vi "AdafruitSeesawNeoPixel.vi"() -> ()   [LabVIEW 2020, in "CTI-Scratchpad.lvlib"]
uses:
  CTI-Scratchpad.lvlib
  CTI/Identity.ctl
  AdafruitSeeSaw/NeoPixelRingPatterns.ctl
  CTI/Error Reporting.ctl
  CTI/I2C Address.ctl
  CTI/GPIO Number.ctl
  CTI/I2C Number.ctl
  CTI/Session/Session.lvclass
  CTI/VisaComms/VisaComms.lvclass
  CTI/CTI.lvlib
  CTI-Peripheral/AdaFruit-Seesaw/AdaFruit-Seesaw.lvclass
panel:
  in  "Timeout":i32=100
  in  "Patterns":T1=enum."ColorWipe"
  in  "Colour Set":T2={"Color Box 0"=16711803, "Color Box 1"=6618880, "Color Box 2"=16716496, "Color Box 4"=9567230, "Color Box 5"=6618880, "Color Box 6"=3381759, "Color Box 7"=9567230, "Color Box 8"=6618880, "Color Box 9"=16860, "Color Box 10"=6618880, "Color Box 11"=6618880, "Color Box 12"=6618880}
  out "NeoPixel Ring":T3={"Color Box"=0, "Color Box 2"=0, "Color Box 3"=0, "Color Box 4"=0, "Color Box 5"=0, "Color Box 6"=0, "Color Box 7"=0, "Color Box 8"=0, "Color Box 9"=0, "Color Box 10"=0, "Color Box 11"=16711680, "Color Box 12"=16777228}
  in  "Brightness":u8=5
  out "loop":i32=14774
  out "Identity":T4
  in  "Grove Connector":enum16{"I2C0", "I2C1"}(ring)
  in  "Port":refnum<visa-resource-name>="COM11"
  out "error out 2":errorcluster
  in  "Stop":bool
  out "error out":errorcluster
  # "https://www.adafruit.com/product/1643"
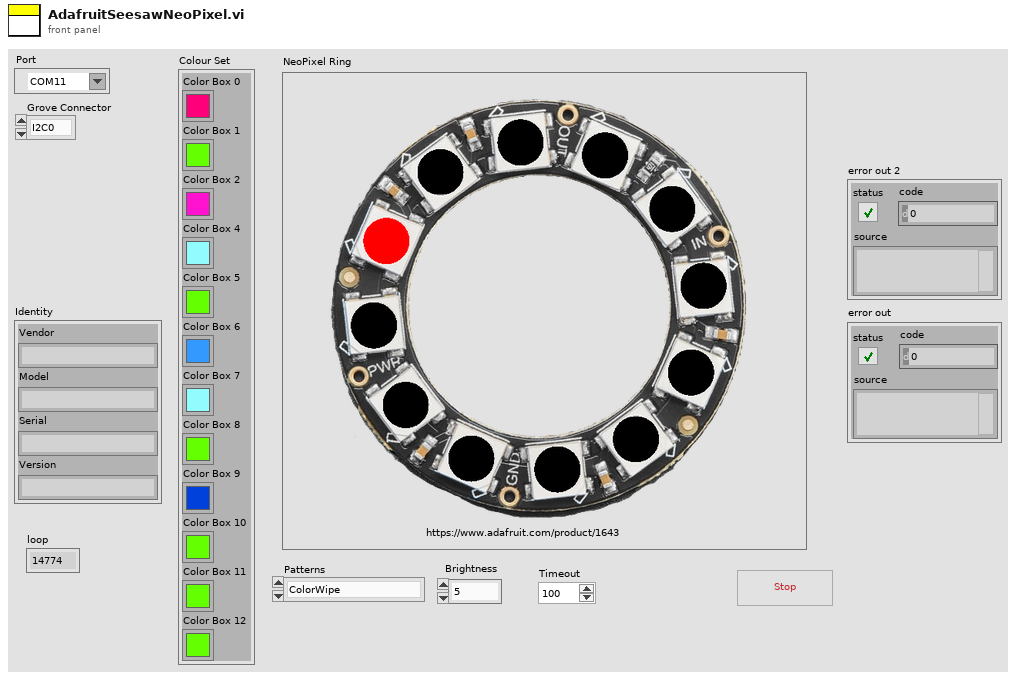
[diagram p1: front panel]
types:
  T1 = typedef "CTI-Scratchpad.lvlib/NeoPixelRingPatterns.ctl" = enum16{"Set Colour", "ColorWipe", "TheatreChase", "Rainbow"}
  T2 = cluster{"Color Box 0":u32, "Color Box 1":u32, "Color Box 2":u32, "Color Box 4":u32, "Color Box 5":u32, "Color Box 6":u32, "Color Box 7":u32, "Color Box 8":u32, "Color Box 9":u32, "Color Box 10":u32, "Color Box 11":u32, "Color Box 12":u32}
  T3 = cluster{"Color Box":u32, "Color Box 2":u32, "Color Box 3":u32, "Color Box 4":u32, "Color Box 5":u32, "Color Box 6":u32, "Color Box 7":u32, "Color Box 8":u32, "Color Box 9":u32, "Color Box 10":u32, "Color Box 11":u32, "Color Box 12":u32}
  T4 = typedef "CTI.lvlib/Identity.ctl" = cluster{"Vendor":string, "Model":string, "Serial":string, "Version":string}
  T5 = cluster{"Color Box 3":u32, "Color Box":u32, "Color Box 2":u32, "Color Box 4":u32, "Color Box 5":u32, "Color Box 6":u32, "Color Box 7":u32, "Color Box 8":u32, "Color Box 9":u32, "Color Box 10":u32, "Color Box 11":u32, "Color Box 12":u32}
  T6 = typedef "CTI.lvlib/I2C Address.ctl" = u8
  T7 = typedef "CTI.lvlib/Error Reporting.ctl" = enum16{"Minimal", "Moderate", "Full"}
  T8 = typedef "CTI.lvlib/I2C Number.ctl" = i8
  T9 = typedef "CTI.lvlib/GPIO Number.ctl" = i8
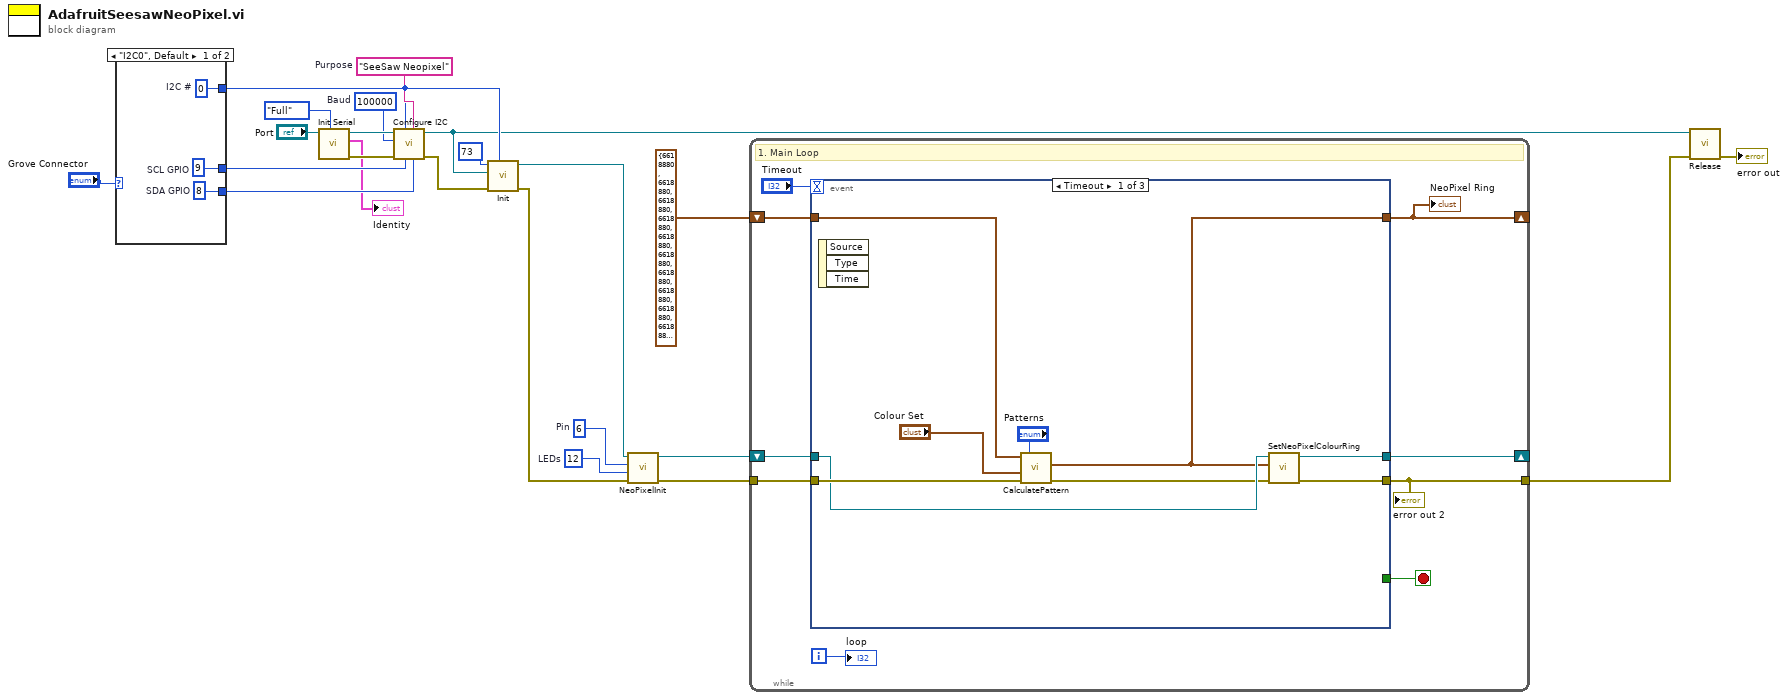
[diagram p0: block diagram]
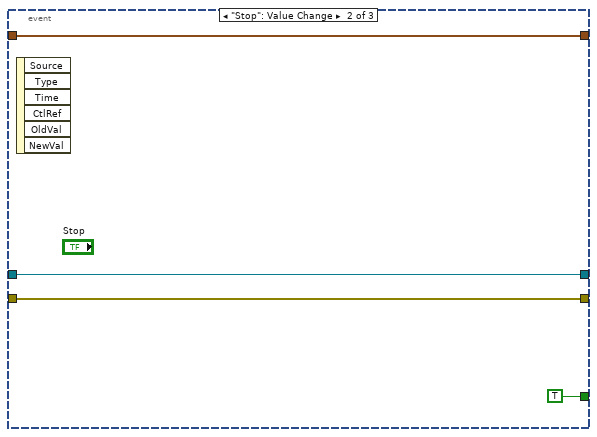
[diagram p2: hidden frame]
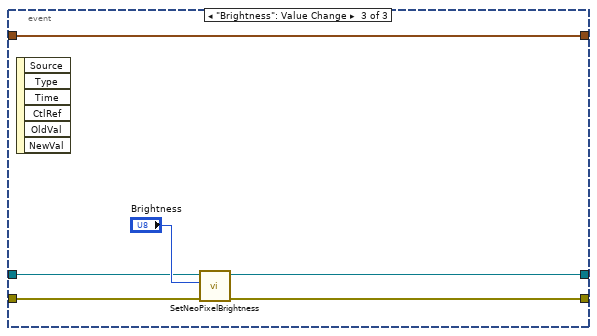
[diagram p3: hidden frame]
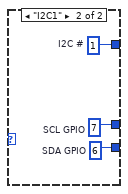
[diagram p4: hidden frame]
diagram:
  w1 = u8 12  # LEDs
  w6 = u8 6  # Pin
  w18 = "SeeSaw Neopixel"  # Purpose
  w19 = u32 100000  # Baud
  n1 = case shown="\"I2C0\", Default" "Grove Connector" {
    tunnel: [w26 w29] -> w16
    tunnel: [w25 w28] -> w15
    tunnel: [w24 w27] -> w11
    frame "I2C0", Default {
      w24 = T8 0  # I2C #
      w25 = T9 8  # SDA GPIO
      w26 = T9 9  # SCL GPIO
    }
    frame "I2C1" {
      w27 = T8 1  # I2C #
      w28 = T9 6  # SDA GPIO
      w29 = T9 7  # SCL GPIO
    }
  }
  n2 = call "Init Serial.vi"("Error Checking (Full)"=Error_Reporting."Full", "VISA resource name in"="Port") -> ("error out"=w20:errorcluster, "Identity"=→"Identity":T4, "Session"=w21:refnum<class "Session.lvclass">)  [unwired: 7 in]
  n3 = call "Configure I2C.vi"("SDA GPIO"=w15, "Purpose (\"I2C\")"=w18, "SCL GPIO"=w16, "I2C #"=w11, "error in (no error)"=w20, "Baud"=w19, "Session in"=w21) -> ("error out"=w9:errorcluster, "Session out"=w10:refnum<class "Session.lvclass">)  [unwired: 3 in]
  n4 = call "Init.vi"("I2C #"=w11, "error in (no error)"=w9, "Session In"=w10, "Address"=T6 73) -> ("error out"=w7:errorcluster, "AdaFruit-Seesaw out"=w8:refnum<class "AdaFruit-Seesaw.lvclass">)  [unwired: 6 in]
  n5 = call "NeoPixelInit.vi"("error in (no error)"=w7, "LEDs"=w1, "Pin"=w6, "AdaFruit-Seesaw in"=w8) -> ("error out"=w3:errorcluster, "AdaFruit-Seesaw out"=w4:refnum<class "AdaFruit-Seesaw.lvclass">)  [unwired: 6 in]
  n6 = while {
    tunnel: w3 -> [w37]
    tunnel: [w35] -> w13
    shift-right: [w33] -> _
    shift-left: w4 -> [w38]
    shift-right: [w31] -> _
    shift-left: T5 {"Color Box 3"=6618880, "Color Box"=6618880, "Color Box 2"=6618880, "Color Box 4"=6618880, "Color Box 5"=6618880, "Color Box 6"=6618880, "Color Box 7"=6618880, "Color Box 8"=6618880, "Color Box 9"=6618880, "Color Box 10"=6618880, "Color Box 11"=6618880, "Color Box 12"=6618880} ("NeoPixel Ring") -> [w32]
    i -> [w36]
    stop <- w34 stop-if-true
    # "1. Main Loop"
    n7 = event shown="[0] Timeout" {
      selector: _ -> [_ _ _]
      dyn-events: _ -> [_ _ _]
      timeout: "Timeout" -> [_ _ _]
      tunnel: w38 -> [w43 w49 w56]
      tunnel: w37 -> [w47 w50 w55]
      tunnel: [w40 w50 w54] -> w35
      tunnel: [_ TRUE _] -> w34
      tunnel: [w41 w49 w53] -> w33
      tunnel: w32 -> [w44 w48 w52]
      tunnel: [w39 w48 w52] -> w31
      event Timeout {
        n8 = event-data() -> ()  [unwired: 1 in, 3 out]
        n9 = call "CalculatePattern.vi"("Patterns"="Patterns", "error in (no error)"=w47, "Colour Set"="Colour Set", "NeoPixel Ring in"=w44) -> ("error out"=w42:errorcluster, "NeoPixel Ring out"=w39:T2)  [unwired: 3 in]
        n10 = call "SetNeoPixelColourRing.vi"("error in (no error)"=w42, "NeoPixel Ring in"=w39, "AdaFruit-Seesaw in"=w43) -> ("error out"=w40:errorcluster, "AdaFruit-Seesaw out"=w41:refnum<class "AdaFruit-Seesaw.lvclass">)  [unwired: 7 in]
      }
      event "Stop": Value Change {
        n11 = event-data() -> ()  [unwired: 1 in, 6 out]
      }
      event "Brightness": Value Change {
        n12 = event-data() -> ()  [unwired: 1 in, 6 out]
        n13 = call "SetNeoPixelBrightness.vi"("error in (no error)"=w55, "Brightness"="Brightness", "AdaFruit-Seesaw in"=w56) -> ("error out"=w54:errorcluster, "AdaFruit-Seesaw out"=w53:refnum<class "AdaFruit-Seesaw.lvclass">)  [unwired: 7 in]
      }
    }
    "error out 2" <- w35
    "NeoPixel Ring" <- w31
    "loop" <- w36
  }
  n14 = call-dynamic "Release.vi"("error in (no error)"=w13, "Session in"=w10) -> ("error out"=→"error out":errorcluster)  [unwired: 9 in]
